vi "4155C Sample Config SMUs v3.0.vi"(4 "Sample - Probe 4":u32(ring)=3 items=["SMU1  ", "SMU2  ", "SMU3  ", "SMU4  ", "SMU5  ", "SMU6  ", "VSU1  ", "VSU2  "], 5 "Sample - Drain":u32(ring)=1 items=["SMU1  ", "SMU2  ", "SMU3  ", "SMU4  ", "SMU5  ", "SMU6  ", "VSU1  ", "VSU2  "], 6 "Sample - Gate":u32(ring)=2 items=["SMU1  ", "SMU2  ", "SMU3  ", "SMU4  ", "SMU5  ", "SMU6  ", "VSU1  ", "VSU2  "], 7 "Sample - Source/Common":u32(ring) items=["SMU1  ", "SMU2  ", "SMU3  ", "SMU4  ", "SMU5  ", "SMU6  ", "VSU1  ", "VSU2  "], 8 "error in (no error)":errorcluster, 9 "Gate Standby":bool, 10 "Drain Standby":bool, 11 "VISA resource name in":refnum<visa-resource-name>) -> (0 "error out":errorcluster, 3 "VISA Resource Name out":refnum<visa-resource-name>)   [LabVIEW 2016]
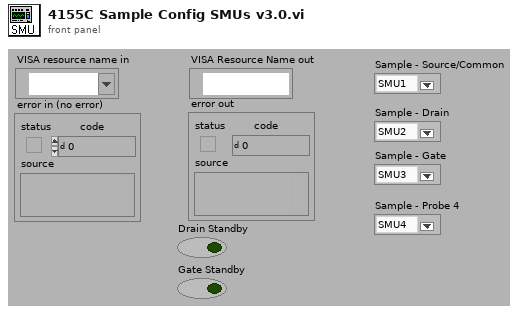
[diagram p1: front panel]
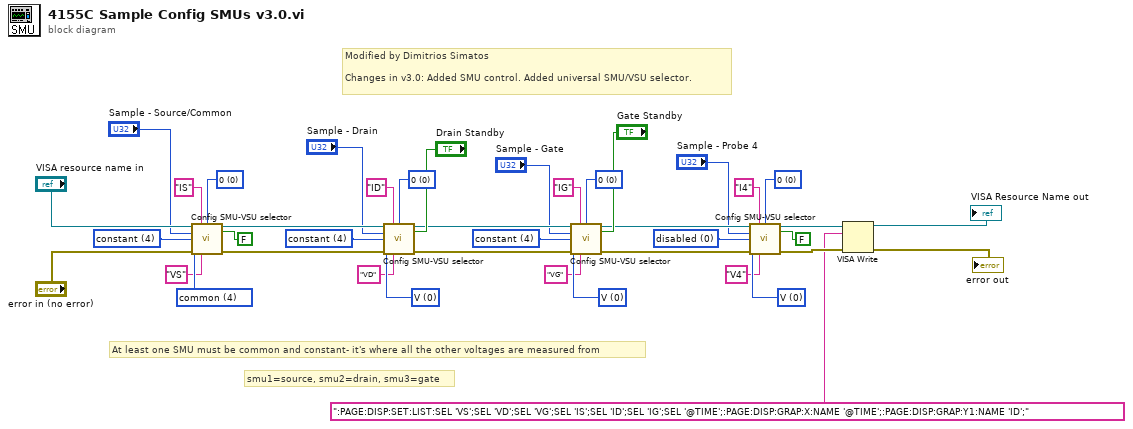
[diagram p0: block diagram]
diagram:
  w18 = u32 0 items=["V  ", "I  ", "V pulse  ", "I pulse  ", "  common  "] ("mode")
  w19 = u32 0 items=["0  ", "10K Ohms  ", "100K Ohms  ", "1M Ohms  "] ("series resistance *")
  w21 = u32 0 items=["disabled  ", "VAR1  ", "VAR2  ", "VAR1'  ", "constant  "] ("function")
  w24 = u32 0 items=["V  ", "I  ", "V pulse  ", "I pulse  ", "  common  "] ("mode")
  w25 = u32 0 items=["0  ", "10K Ohms  ", "100K Ohms  ", "1M Ohms  "] ("series resistance *")
  w27 = u32 4 items=["disabled  ", "VAR1  ", "VAR2  ", "VAR1'  ", "constant  "] ("function")
  w30 = u32 0 items=["V  ", "I  ", "V pulse  ", "I pulse  ", "  common  "] ("mode")
  w31 = u32 0 items=["0  ", "10K Ohms  ", "100K Ohms  ", "1M Ohms  "] ("series resistance *")
  w33 = u32 4 items=["disabled  ", "VAR1  ", "VAR2  ", "VAR1'  ", "constant  "] ("function")
  w36 = u32 4 items=["V  ", "I  ", "V pulse  ", "I pulse  ", "  common  "] ("mode")
  w37 = u32 0 items=["0  ", "10K Ohms  ", "100K Ohms  ", "1M Ohms  "] ("series resistance *")
  w39 = u32 4 items=["disabled  ", "VAR1  ", "VAR2  ", "VAR1'  ", "constant  "] ("function")
  # "Modified by Dimitrios Simatos\n\nChanges in v3.0: Added SMU control. Added universal SMU/VSU selector."
  # "smu1=source, smu2=drain, smu3=gate"
  # "At least one SMU must be common and constant- it's where all the other voltages are measured from"
  n1 = call "Config SMU-VSU selector.vi"("VISA session"="VISA resource name in", "I name (max 6 chars)"="IS", "standby"=FALSE, "unit to configure"="Sample - Source/Common", "function"=w39, "mode"=w36, "error in (no error)"="error in (no error)", "V name (max 6 chars)"="VS", "series resistance *"=w37) -> ("dup VISA resource name"=w15:refnum<visa-resource-name>, "error out"=w14:errorcluster)  [unwired: 3 in, 2 out]
  n2 = call "Config SMU-VSU selector.vi"("VISA session"=w15, "I name (max 6 chars)"="ID", "standby"="Drain Standby", "unit to configure"="Sample - Drain", "function"=w33, "mode"=w30, "error in (no error)"=w14, "V name (max 6 chars)"="VD", "series resistance *"=w31) -> ("dup VISA resource name"=w12:refnum<visa-resource-name>, "error out"=w13:errorcluster)  [unwired: 3 in, 2 out]
  n3 = call "Config SMU-VSU selector.vi"("VISA session"=w12, "I name (max 6 chars)"="IG", "standby"="Gate Standby", "unit to configure"="Sample - Gate", "function"=w27, "mode"=w24, "error in (no error)"=w13, "V name (max 6 chars)"="VG", "series resistance *"=w25) -> ("dup VISA resource name"=w11:refnum<visa-resource-name>, "error out"=w10:errorcluster)  [unwired: 3 in, 2 out]
  n4 = call "Config SMU-VSU selector.vi"("VISA session"=w11, "I name (max 6 chars)"="I4", "standby"=FALSE, "unit to configure"="Sample - Probe 4", "function"=w21, "mode"=w18, "error in (no error)"=w10, "V name (max 6 chars)"="V4", "series resistance *"=w19) -> ("dup VISA resource name"=w9:refnum<visa-resource-name>, "error out"=w8:errorcluster)  [unwired: 3 in, 2 out]
  n5 = VISA Write(VISA resource name=w9, write buffer=":PAGE:DISP:SET:LIST:SEL 'VS';SEL 'VD';SEL 'VG';SEL 'IS';SEL 'ID';SEL 'IG';SEL '@TIME';:PAGE:DISP:GRAP:X:NAME '@TIME';:PAGE:DISP:GRAP:Y1:NAME 'ID';" ("write buffer (\"\")"), error in (no error)=w8) -> (VISA resource name out=→"VISA Resource Name out":refnum<visa-resource-name>, error out=→"error out":errorcluster)  [unwired: 1 out]
